vi "util-collect-error.vi"(10 "error in (no error)":errorcluster, 11 "Array in":errorcluster[](array[cluster])) -> (3 "Array out":errorcluster[](array[cluster]))   [LabVIEW 2024]
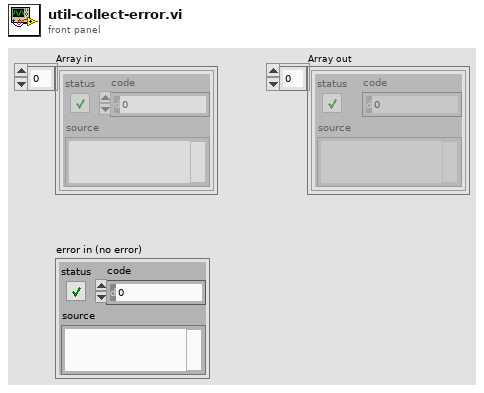
[diagram p1: front panel]
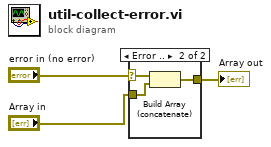
[diagram p0: block diagram]
diagram:
  n1 = case shown="Error .." "error in (no error)" {
    selector: "error in (no error)" -> [_ w5]
    tunnel: [w4 w7] -> w1
    tunnel: "Array in" -> [w4 w6]
    frame No Error {
    }
    frame Error {
      n2 = Build Array (concatenate)(w5, w6) -> (w7:errorcluster[])
    }
  }
  "Array out" <- w1
